vi "Actor Core.vi"(8 "error in":errorcluster, 11 "Executive View In":refnum<class "Executive View.lvclass">) -> (0 "error out":errorcluster, 3 "Actor out":refnum<class "Actor.lvclass">)   [LabVIEW 2017, in "Executive View.lvlib" / "Executive View.lvclass"]
uses:
  <vilib>/gpm_packages/TestSystem/Views/Executive View/Executive View/Executive View.lvclass
  <vilib>/ActorFramework/Actor/Actor.lvclass
  <vilib>/gpm_packages/@cs/mva-viewable/Source/IViewable/IViewable/IViewable.lvclass
panel:
  in  "Executive View":i32(listbox)
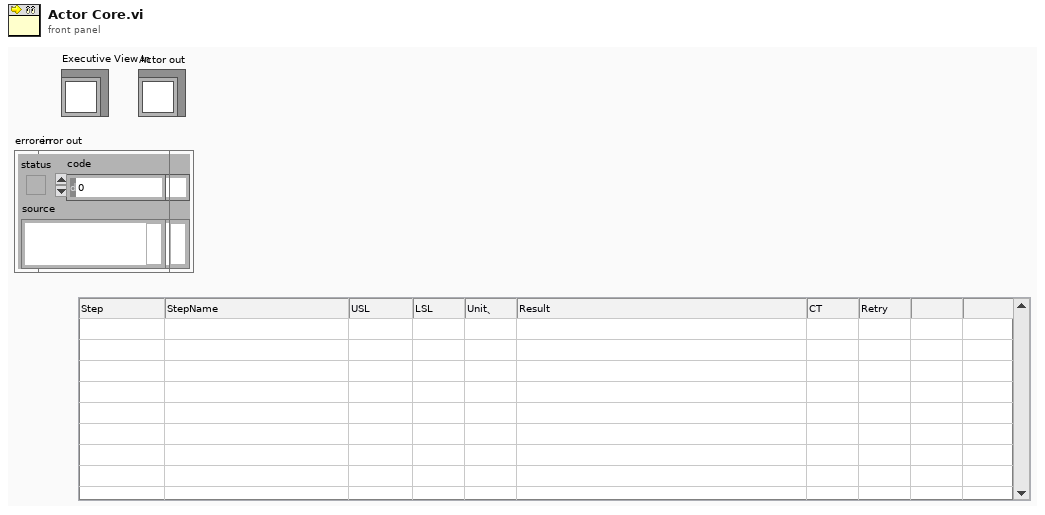
[diagram p1: front panel]
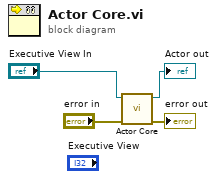
[diagram p0: block diagram]
diagram:
  n1 = call-parent "Actor Core.vi"("error in"="error in", "IViewable In"="Executive View In") -> ("error out"=→"error out":errorcluster, "Actor out"=→"Actor out":refnum<class "Actor.lvclass">)  [unwired: 8 in]
